vi "Pico5000 - AdcToVolts.vi"(0 "Max ADC":i16=32767, 2 "Range Index":u16, 3 "Data":i16[](array[numeric])) -> (1 "Data (Volts)":dbl[](array[numeric]))   [LabVIEW 2016]
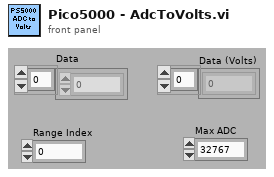
[diagram p1: front panel]
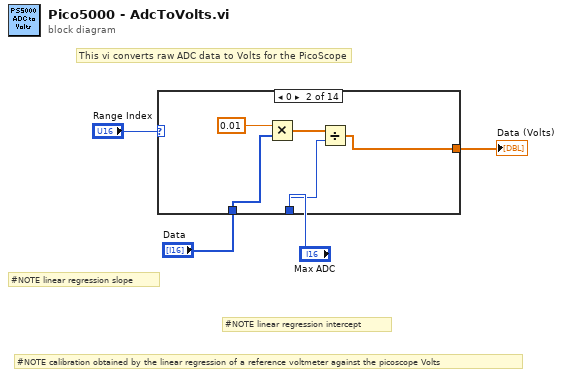
[diagram p0: block diagram]
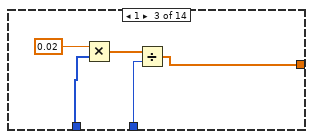
[diagram p3: hidden frame]
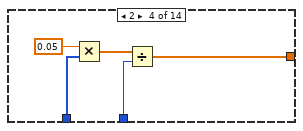
[diagram p4: hidden frame]
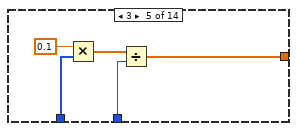
[diagram p5: hidden frame]
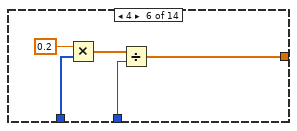
[diagram p6: hidden frame]
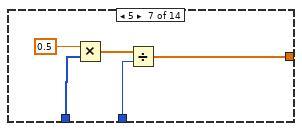
[diagram p7: hidden frame]
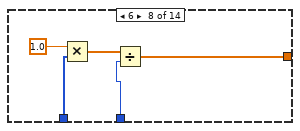
[diagram p8: hidden frame]
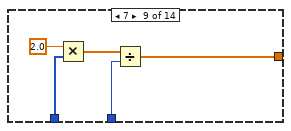
[diagram p9: hidden frame]
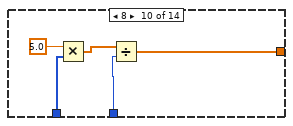
[diagram p10: hidden frame]
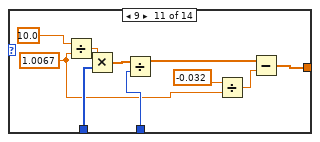
[diagram p11: hidden frame]
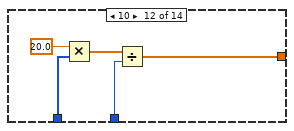
[diagram p12: hidden frame]
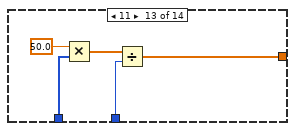
[diagram p13: hidden frame]
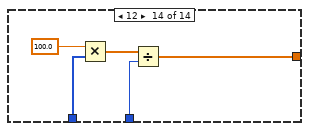
[diagram p14: hidden frame]
diagram:
  # "#NOTE calibration obtained by the linear regression of a reference voltmeter against the picoscope Volts"
  # "#NOTE linear regression intercept"
  # "#NOTE linear regression slope"
  # "This vi converts raw ADC data to Volts for the PicoScope"
  n1 = case shown="0" "Range Index" {
    tunnel: [w5 w8 w11 w18 w23 w28 w33 w37 w43 w48 w54 w63 w68 w73] -> w2
    tunnel: "Data" -> [w5 w7 w13 w17 w22 w27 w32 w38 w42 w47 w59 w62 w67 w72]
    tunnel: "Max ADC" -> [_ w6 w12 w16 w21 w26 w31 w36 w41 w46 w58 w61 w66 w71]
    frame Default {
    }
    frame 0 {
      n2 = Multiply(x=0.01, y=w7) -> (x*y=w10:dbl[])
      n3 = Divide(x=w10, y=w6) -> (x/y=w8:dbl[])
    }
    frame 1 {
      n4 = Multiply(x=0.02, y=w13) -> (x*y=w15:dbl[])
      n5 = Divide(x=w15, y=w12) -> (x/y=w11:dbl[])
    }
    frame 2 {
      n6 = Multiply(x=0.05, y=w17) -> (x*y=w19:dbl[])
      n7 = Divide(x=w19, y=w16) -> (x/y=w18:dbl[])
    }
    frame 3 {
      n8 = Multiply(x=0.1, y=w22) -> (x*y=w24:dbl[])
      n9 = Divide(x=w24, y=w21) -> (x/y=w23:dbl[])
    }
    frame 4 {
      n10 = Multiply(x=0.2, y=w27) -> (x*y=w30:dbl[])
      n11 = Divide(x=w30, y=w26) -> (x/y=w28:dbl[])
    }
    frame 5 {
      n12 = Multiply(x=0.5, y=w32) -> (x*y=w35:dbl[])
      n13 = Divide(x=w35, y=w31) -> (x/y=w33:dbl[])
    }
    frame 6 {
      n14 = Multiply(x=1.0, y=w38) -> (x*y=w40:dbl[])
      n15 = Divide(x=w40, y=w36) -> (x/y=w37:dbl[])
    }
    frame 7 {
      n16 = Multiply(x=2.0, y=w42) -> (x*y=w45:dbl[])
      n17 = Divide(x=w45, y=w41) -> (x/y=w43:dbl[])
    }
    frame 8 {
      n18 = Multiply(x=5.0, y=w47) -> (x*y=w50:dbl[])
      n19 = Divide(x=w50, y=w46) -> (x/y=w48:dbl[])
    }
    frame 9 {
      w51 = 1.0067 ("x")
      n20 = Divide(x=10.0, y=w51) -> (x/y=w57:dbl)
      n21 = Multiply(x=w57, y=w59) -> (x*y=w60:dbl[])
      n22 = Divide(x=w60, y=w58) -> (x/y=w55:dbl[])
      n23 = Divide(x=-0.032, y=w51) -> (x/y=w53:dbl)
      n24 = Subtract(x=w55, y=w53) -> (x-y=w54:dbl[])
    }
    frame 10 {
      n25 = Multiply(x=20.0, y=w62) -> (x*y=w65:dbl[])
      n26 = Divide(x=w65, y=w61) -> (x/y=w63:dbl[])
    }
    frame 11 {
      n27 = Multiply(x=50.0, y=w67) -> (x*y=w70:dbl[])
      n28 = Divide(x=w70, y=w66) -> (x/y=w68:dbl[])
    }
    frame 12 {
      n29 = Multiply(x=100.0, y=w72) -> (x*y=w75:dbl[])
      n30 = Divide(x=w75, y=w71) -> (x/y=w73:dbl[])
    }
  }
  "Data (Volts)" <- w2
